vi "DeleteRobotByID.vi"(8 "error in (no error)":errorcluster, 9 "id":i32, 10 "RobotRef":refnum<class "Robot.lvclass">[](array[class]), 11 "Utilities in":refnum<class "Utilities.lvclass">) -> (0 "error out":errorcluster, 2 "RobotRef out":refnum<class "Robot.lvclass">[](array[class]), 3 "Utilities out":refnum<class "Utilities.lvclass">)   [LabVIEW 2023, in "Utilities.lvclass"]
uses:
  Utilities.lvclass
  Robot_class/Robot.lvclass
  Robot_class/Robot.lvclass/Robot.ctl
  Robot_class/Read id.vi
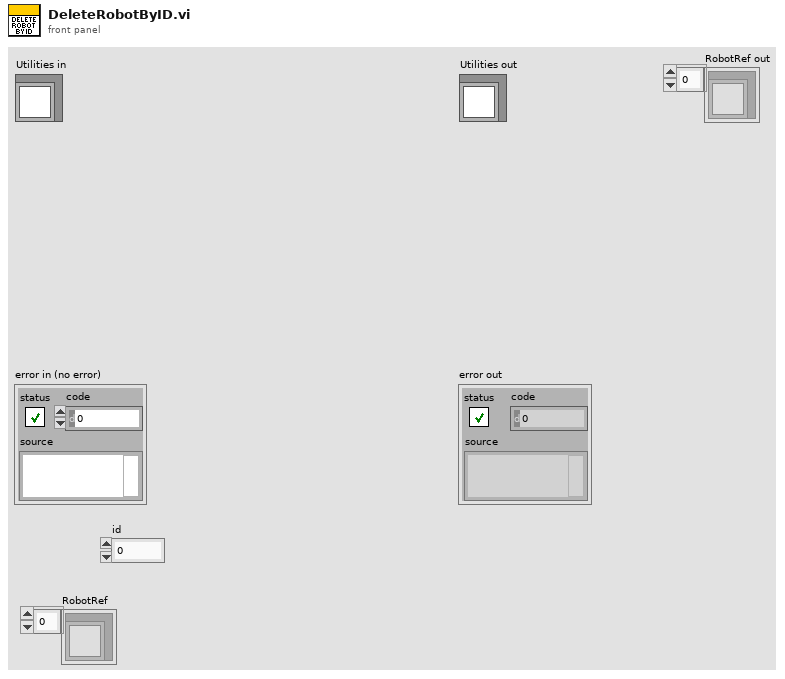
[diagram p1: front panel]
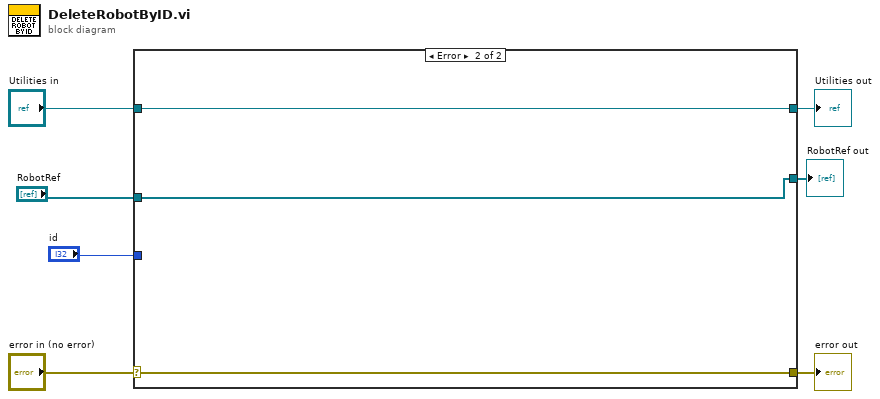
[diagram p0: block diagram]
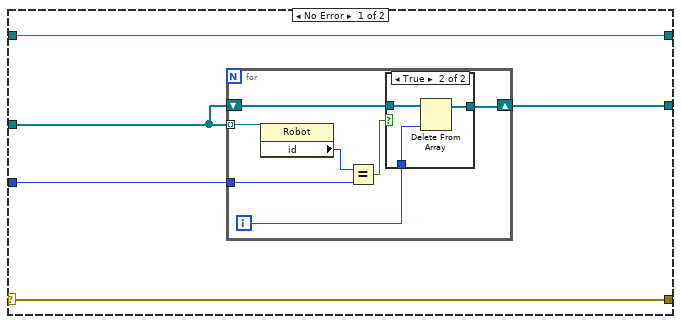
[diagram p2: hidden frame]
diagram:
  n1 = case shown="Error" "error in (no error)" {
    selector: "error in (no error)" -> [w11 w26]
    tunnel: [w11 w26] -> w6
    tunnel: [w12 w25] -> w4
    tunnel: "Utilities in" -> [w12 w25]
    tunnel: "RobotRef" -> [w9 w24]
    tunnel: "id" -> [w10 _]
    tunnel: [w8 w24] -> w1
    frame No Error {
      n2 = for {
        tunnel: w9 -> [w19] mode=indexing
        tunnel: w10 -> [w17]
        shift-right: [w14] -> w8
        shift-left: w9 -> [w16]
        i -> [w15]
        n3 = property class="Robot"(reference=w19) -> ("id"=w18:i32)  [unwired: 1 in, 2 out]
        n4 = Equal?(x=w18, y=w17) -> (x = y?=w13:bool)
        n5 = case shown="True" w13 {
          tunnel: w16 -> [w20 w23]
          tunnel: w15 -> [_ w22]
          tunnel: [w20 w21] -> w14
          frame False {
          }
          frame True {
            n6 = Delete From Array(array=w23, index=w22) -> (array with subset deleted=w21:refnum<class "Robot.lvclass">[])  [unwired: 1 in, 1 out]
          }
        }
      }
    }
    frame Error {
    }
  }
  "error out" <- w6
  "Utilities out" <- w4
  "RobotRef out" <- w1
